vi "HttpPost.vi"(6 "request specific headers":T1[](array[typedef]), 7 "binary string":bool, 8 "error in":errorcluster, 9 "body":string, 10 "url":string, 11 "reQwestClient in":refnum<class "reQwestClient.lvclass">) -> (0 "error out":errorcluster, 1 "headers":cluster{"name":string, "value":string}[](array[cluster]), 2 "response_body":string, 3 "reQwestClient out":refnum<class "reQwestClient.lvclass">)   [LabVIEW 2020, in "reQwestClient.lvclass"]
uses:
  reQwestClient.lvclass
  <vilib>/addons/_JKI.lib/REST Client/classes/REST Client/HTTP Header.ctl
  submodules/reqwest-rs-labview/lv_src/Types/http_method_enum.ctl
  reQwestClient.lvclass/reQwestClient.ctl
  submodules/reqwest-rs-labview/lv_src/Request/Request.lvclass
  submodules/reqwest-rs-labview/lv_src/Client/Client.lvclass
  submodules/reqwest-rs-labview/lv_src/reqwest.lvlib
  submodules/reqwest-rs-labview/lv_src/RequestBuilder/RequestBuilder.lvclass
  submodules/reqwest-rs-labview/lv_src/Headers/Headers.lvclass
  <vilib>/addons/_JKI.lib/REST Client/classes/REST Client/REST Client.lvclass
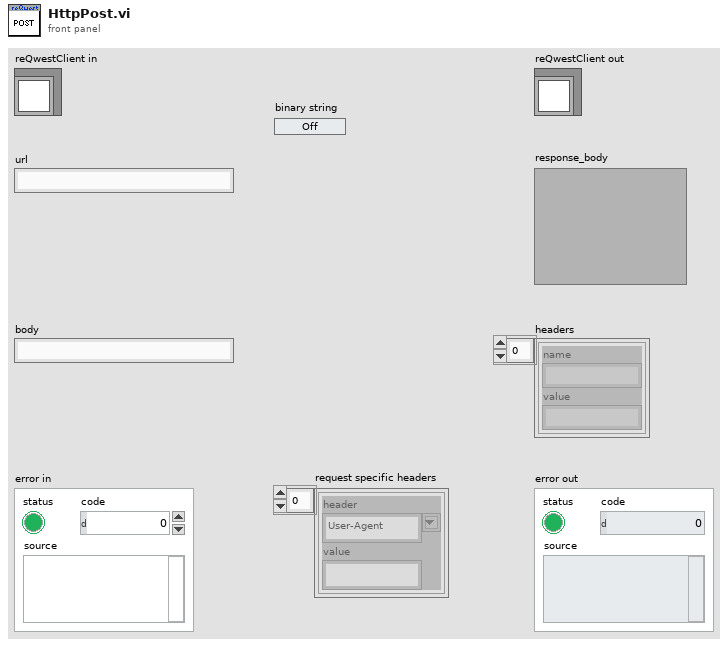
[diagram p1: front panel]
types:
  T1 = typedef "REST Client.lvlib/REST Client.lvclass/HTTP Header.ctl" = cluster{"header":string, "value":string}
  T2 = typedef "reqwest.lvlib/http_method_enum.ctl" = enum8{"<select>", "GET", "POST", "PUT", "DELETE", "HEAD", "OPTIONS", "CONNECT", "PATCH", "TRACE"}
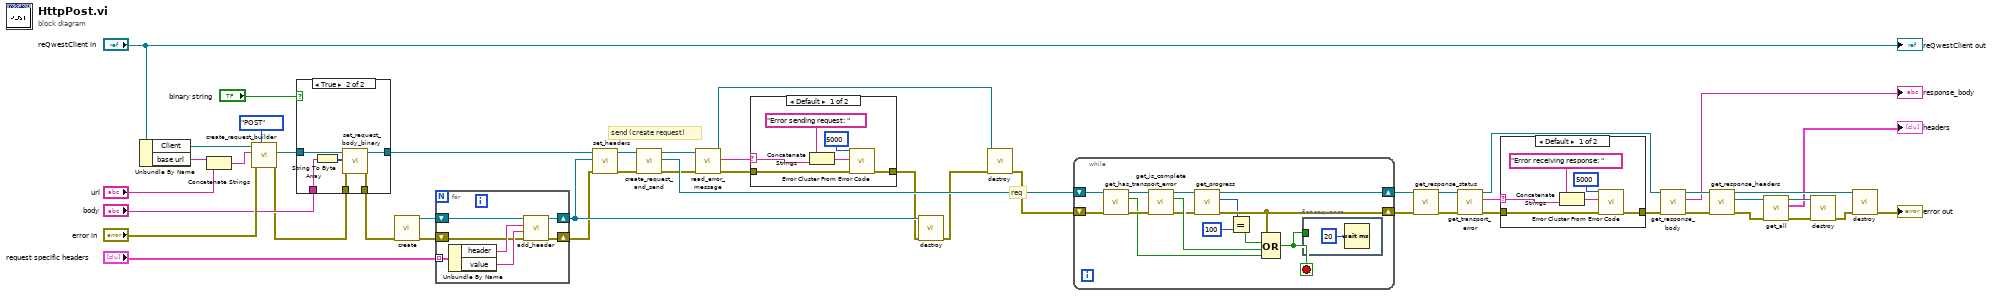
[diagram p0: block diagram]
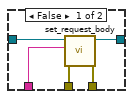
[diagram p2: hidden frame]
diagram:
  # "send (create request)"
  # "req"
  n1 = Unbundle By Name("reQwestClient in") -> ("Client"=w29:refnum<class "Client.lvclass">, "base url"=w17:string)
  n2 = Concatenate Strings(w17, "url") -> (w15:string)
  n3 = call "create_request_builder.vi"("HTTP Method"=http_method_enum."POST", "error in (no error)"="error in", "url"=w15, "Client in"=w29) -> ("error out"=w4:errorcluster, "RequestBuilder out"=w7:refnum<class "RequestBuilder.lvclass">)  [unwired: 5 in, 1 out]
  n4 = case shown="True" "binary string" {
    tunnel: w7 -> [w53 w59]
    tunnel: "body" -> [w52 w55]
    tunnel: [w51 w58] -> w5
    tunnel: w4 -> [w50 w56]
    tunnel: [w49 w57] -> w3
    frame False {
      n5 = call "set_request_body.vi"("error in"=w50, "body"=w52, "obj in"=w53) -> ("error out"=w49:errorcluster, "obj out"=w51:refnum<class "RequestBuilder.lvclass">)  [unwired: 6 in, 1 out]
    }
    frame True {
      n6 = String To Byte Array(string=w55) -> (unsigned byte array=w54:u8[])
      n7 = call "set_request_body_binary.vi"("error in"=w56, "binary body"=w54, "obj in"=w59) -> ("error out"=w57:errorcluster, "obj out"=w58:refnum<class "RequestBuilder.lvclass">)  [unwired: 6 in, 1 out]
    }
  }
  n8 = call "create.vi"("error in (no error)"=w3) -> ("error out"=w26:errorcluster, "Headers out"=w28:refnum<class "Headers.lvclass">)  [unwired: 9 in]
  n9 = for {
    tunnel: "request specific headers" -> [w65] mode=indexing
    shift-right: [w61] -> w23
    shift-left: w28 -> [w66]
    shift-right: [w60] -> w21
    shift-left: w26 -> [w62]
    n10 = Unbundle By Name(w65) -> ("header"=w64:string, "value"=w63:string)
    n11 = call "add_header.vi"("error in (no error)"=w62, "value"=w63, "key"=w64, "Headers in"=w66) -> ("error out"=w60:errorcluster, "Headers out"=w61:refnum<class "Headers.lvclass">)  [unwired: 5 in, 1 out]
  }
  n12 = call "set_headers.vi"("error in (no error)"=w21, "Headers"=w23, "obj in"=w5) -> ("error out"=w24:errorcluster, "obj out"=w25:refnum<class "RequestBuilder.lvclass">)  [unwired: 6 in, 1 out]
  n13 = call "create_request_and_send.vi"("error in"=w24, "obj in"=w25) -> ("error out"=w32:errorcluster, "request"=w35:refnum<class "Request.lvclass">, "obj out"=w33:refnum<class "RequestBuilder.lvclass">)  [unwired: 7 in]
  n14 = call "read_error_message.vi"("error in (no error)"=w32, "RequestBuilder in"=w33) -> ("error out"=w14:errorcluster, "error_message"=w12:string, "RequestBuilder in"=w34:refnum<class "RequestBuilder.lvclass">)  [unwired: 7 in]
  n15 = case shown="Default" w12 {
    selector: w12 -> [w69 _]
    tunnel: w14 -> [w72 w73]
    tunnel: [w71 w73] -> w13
    frame Default {
      n16 = Concatenate Strings("Error sending request: " ("error message (\"\")"), w69) -> (w70:string)
      n17 = call <vilib>:"Error Cluster From Error Code.vi"("error in (no error)"=w72, "error message (\"\")"=w70, "error code (0)"=5000) -> ("error out"=w71:errorcluster)  [unwired: 6 in]
    }
    frame "" {
    }
  }
  n18 = call "destroy.vi"("error in (no error)"=w13, "Headers in"=w23) -> ("error out"=w22:errorcluster)  [unwired: 9 in]
  n19 = call "destroy.vi"("error in"=w22, "RequestBuilder in"=w34) -> ("error out"=w31:errorcluster)  [unwired: 8 in, 1 out]
  n20 = while {
    shift-right: [w85] -> w39
    shift-left: w35 -> [w78]
    shift-right: [w83] -> w38
    shift-left: w31 -> [w77]
    stop <- w79 stop-if-true
    n21 = call "get_has_transport_error.vi"("error in (no error)"=w77, "Request in"=w78) -> ("error out"=w75:errorcluster, "has_transport_error"=w74:bool, "Request out"=w76:refnum<class "Request.lvclass">)  [unwired: 7 in]
    n22 = call "get_is_complete.vi"("error in (no error)"=w75, "Request in"=w76) -> ("error out"=w84:errorcluster, "is_complete"=w87:bool, "Request out"=w86:refnum<class "Request.lvclass">)  [unwired: 7 in]
    n23 = call "get_progress.vi"("error in (no error)"=w84, "Request in"=w86) -> ("error out"=w83:errorcluster, "progress"=w81:i32, "Request out"=w85:refnum<class "Request.lvclass">)  [unwired: 7 in]
    n24 = Equal?(x=w81, y=100 ("progress")) -> (x = y?=w80:bool)
    n25 = Compound Arithmetic op=OR(w83, w80, w87, w74) -> (w79:bool)
    n26 = flat-sequence {
      tunnel: w79 -> [_]
      frame #0 {
        n27 = Wait (ms)(milliseconds to wait=u32 20) -> ()  [unwired: 1 out]
      }
    }
  }
  n28 = call "get_response_status.vi"("error in (no error)"=w38, "Request in"=w39) -> ("error out"=w37:errorcluster, "Request out"=w36:refnum<class "Request.lvclass">)  [unwired: 7 in, 1 out]
  n29 = call "get_transport_error.vi"("error in (no error)"=w37, "Request in"=w36) -> ("error out"=w10:errorcluster, "transport_error"=w11:string, "Request in"=w8:refnum<class "Request.lvclass">)  [unwired: 7 in]
  n30 = case shown="Default" w11 {
    selector: w11 -> [w91 _]
    tunnel: w10 -> [w94 w95]
    tunnel: [w93 w95] -> w9
    frame Default {
      n31 = Concatenate Strings("Error receiving response: " ("error message (\"\")"), w91) -> (w92:string)
      n32 = call <vilib>:"Error Cluster From Error Code.vi"("error in (no error)"=w94, "error message (\"\")"=w92, "error code (0)"=5000) -> ("error out"=w93:errorcluster)  [unwired: 6 in]
    }
    frame "" {
    }
  }
  n33 = call "get_response_body.vi"("error in (no error)"=w9, "Request in"=w8) -> ("error out"=w45:errorcluster, "string_value"=→"response_body":string, "Request in"=w47:refnum<class "Request.lvclass">)  [unwired: 7 in]
  n34 = call "get_response_headers.vi"("error in (no error)"=w45, "Request in"=w47) -> ("error out"=w43:errorcluster, "response_headers"=w44:refnum<class "Headers.lvclass">, "Request in"=w46:refnum<class "Request.lvclass">)  [unwired: 7 in]
  n35 = call "get_all.vi"("error in (no error)"=w43, "Headers in"=w44) -> ("error out"=w41:errorcluster, "headers"=→"headers":cluster{"name":string, "value":string}[], "Headers in"=w42:refnum<class "Headers.lvclass">)  [unwired: 6 in, 1 out]
  n36 = call "destroy.vi"("error in (no error)"=w41, "Headers in"=w42) -> ("error out"=w40:errorcluster)  [unwired: 9 in]
  n37 = call "destroy.vi"("error in (no error)"=w40, "Request in"=w46) -> ("error out"=→"error out":errorcluster)  [unwired: 8 in, 1 out]
  "reQwestClient out" <- "reQwestClient in"
